vi "nirviLrmPalette_MergeVI_Memory.vi"   [LabVIEW 2017]
doc: "Represents a VI-defined memory item. Right-click the node and select <B>Configure</B> to configure the VI-defined memory item."
uses:
  <vilib>/rvi/DataTransferAndStorage/Container/Common/niFpgaContainerGetUniqueNameForEmu.vi
  <vilib>/rvi/DataTransferAndStorage/Container/Common/niFpgaContainerSetEmuInfo.vi
  <vilib>/rvi/eio/common/nirviEmuReportErrorAndStop.vi
  <vilib>/rvi/LocalResourceManager/LocalResourceManager.xnode
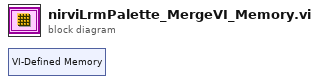
[diagram p0: block diagram]
diagram:
  n1 = xnode "VI-Defined Memory"() -> ()  [unwired: 1 out]
